vi "Render.vi"(8 "error in (no error)":errorcluster, 10 "String in":string, 11 "LineBreak in":refnum<class "LineBreak.lvclass">) -> (0 "error out":errorcluster, 2 "String out":string, 3 "LineBreak out":refnum<class "LineBreak.lvclass">)   [LabVIEW 2021, in "Markdown.lvlib" / "LineBreak.lvclass"]
uses:
  LineBreak.lvclass
  GetBreakTag.vi
  LineBreak.lvclass/LineBreak.ctl
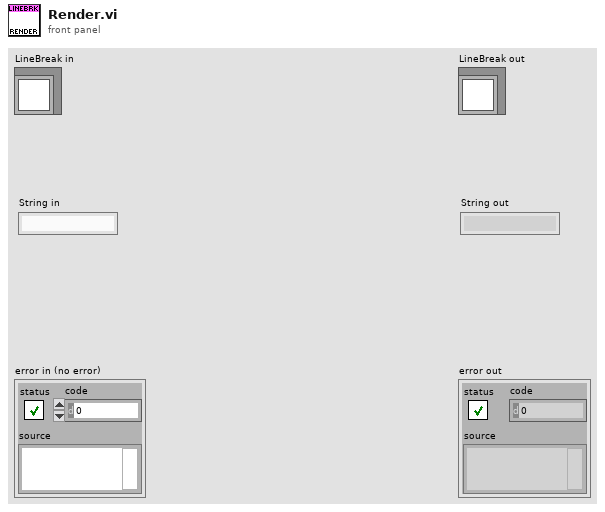
[diagram p1: front panel]
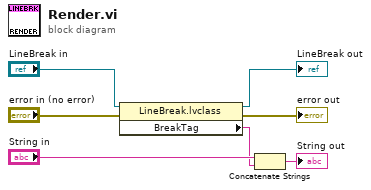
[diagram p0: block diagram]
diagram:
  n1 = property class="LineBreak.lvclass"(reference="LineBreak in", error in="error in (no error)") -> (reference out=→"LineBreak out":refnum<class "LineBreak.lvclass">, error out=→"error out":errorcluster, "BreakTag"=w1:string)
  n2 = Concatenate Strings("String in", w1) -> (→"String out":string)
